vi "dT.vi"() -> (3 "Period":dbl format="%#_6f")   [LabVIEW 2020, in "DAQ AO SFP.lvlib"]
uses:
  DAQ AO SFP.lvlib
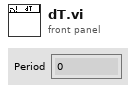
[diagram p1: front panel]
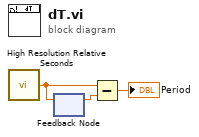
[diagram p0: block diagram]
diagram:
  n1 = call <vilib>:"High Resolution Relative Seconds.vi"() -> ("relative seconds"=w1:dbl)
  n2 = feedback #1() -> (w2:dbl)  [unwired: 1 in]
  n3 = feedback-in #1(w1) -> ()
  n4 = Subtract(x=w1, y=w2) -> (x-y=→"Period":dbl)
